vi "options.vi"(10 "application request in":T4, 11 "test responder in":refnum<class "test responder.lvclass">) -> (2 "application response out":T1, 3 "test responder out":refnum<class "test responder.lvclass">)   [LabVIEW 2016, in "test responder.lvclass"]
uses:
  test responder.lvclass
  http/HTTP server/http request.ctl
  http/HTTP server/http method.ctl
  http/HTTP server/http header data.ctl
  http/HTTP server/http response.ctl
  http/HTTP server/http response packet type.ctl
  http/HTTP responder/http responder.lvclass
  http/HTTP server/Basic HTTP server.lvclass
  http/HTTP server/headers/http headers.lvlib
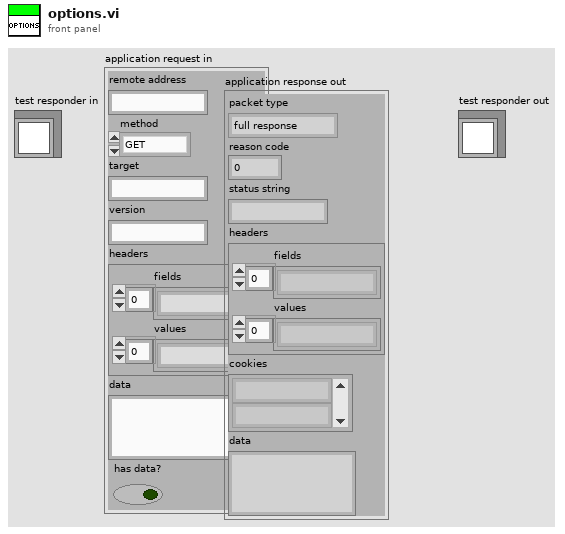
[diagram p1: front panel]
types:
  T1 = typedef "Basic HTTP server.lvclass/http response.ctl" = cluster{"packet type":T2, "reason code":u16, "status string":string, "headers":T3, "cookies":string[], "data":string}
  T2 = typedef "Basic HTTP server.lvclass/http response packet type.ctl" = enum16{"full response", "header only", "data only", "last data"}
  T3 = typedef "http headers.lvlib/http header data.ctl" = cluster{"fields":string[], "values":string[]}
  T4 = typedef "Basic HTTP server.lvclass/http request.ctl" = cluster{"remote address":string, "method":T5, "target":string, "version":string, "headers":T3, "data":string, "has data?":bool}
  T5 = typedef "Basic HTTP server.lvclass/http method.ctl" = enum16{"GET", "POST", "PUT", "DELETE", "HEAD", "OPTIONS", "upgrade"}
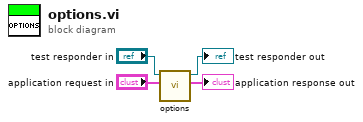
[diagram p0: block diagram]
diagram:
  n1 = call-parent "options.vi"("application request in"="application request in", "http responder in"="test responder in") -> ("application response out"=→"application response out":T1, "http responder out"=→"test responder out":refnum<class "test responder.lvclass">)  [unwired: 8 in]
